vi "MotorDrehzahlerMittlung.vi"() -> ()   [LabVIEW 2019]
uses:
  <vilib>/Analysis/2dsp.llb/Real FFT.vi
  <vilib>/Analysis/NI_AALPro.lvlib
panel:
  out "Amplitude":dbl[](graph)
  out "Phase":dbl[](graph)
  out "Sawtooth":dynamicdata(graph)
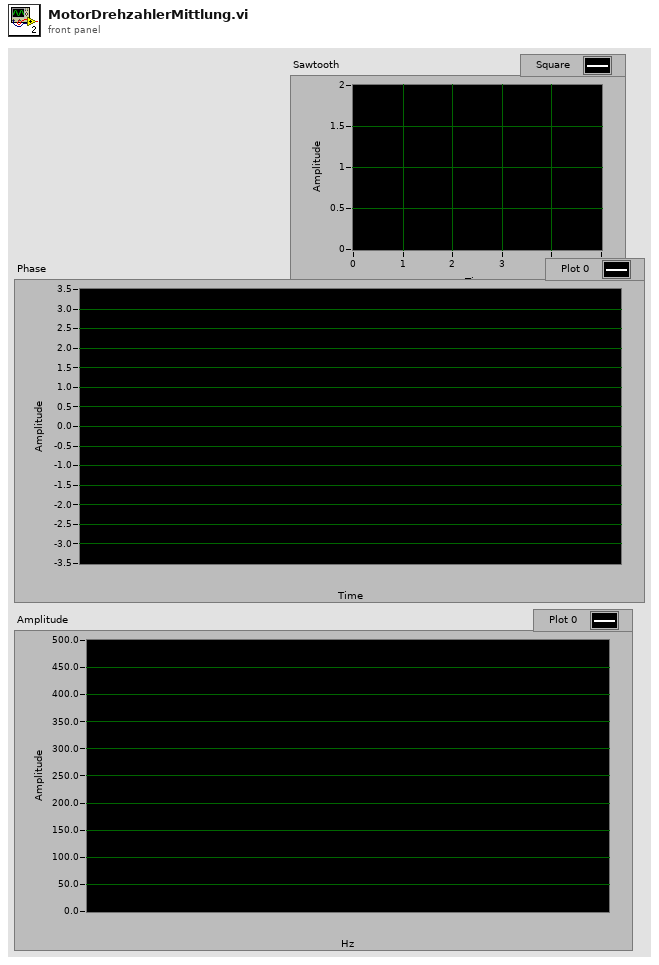
[diagram p1: front panel]
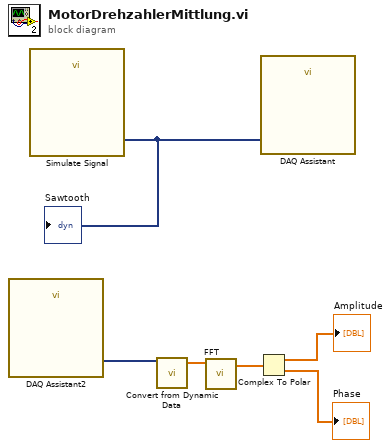
[diagram p0: block diagram]
diagram:
  n1 = call "DAQ Assistant2"() -> ("data"=w2:dynamicdata)  [unwired: 17 in, 2 out]
  n2 = call "Simulate Signal"() -> ("Square"=w6:dynamicdata)  [unwired: 14 in, 1 out]
  "Sawtooth" <- w6
  n3 = call "Convert from Dynamic Data"("Dynamic Data Type"=w2) -> ("Array"=w1:dbl[])  [unwired: 3 in]
  n4 = call-poly <vilib>:"FFT.vi"("X"=w1) -> ("FFT {X}"=w5:cdb[])  [unwired: 9 in, 1 out]
  n5 = Complex To Polar(r * e^(i*theta)=w5) -> (r=→"Amplitude":dbl[], theta=→"Phase":dbl[])
  n6 = call "DAQ Assistant"("data"=w6) -> ()  [unwired: 17 in, 2 out]
